vi "convertChannel.vi"(1 "Chn in":string) -> (0 "Chn out":string)   [LabVIEW 2023, in "ScopeNi.lvclass"]
uses:
  ScopeNi.lvclass
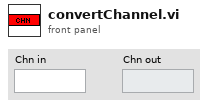
[diagram p1: front panel]
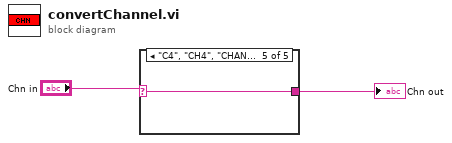
[diagram p0: block diagram]
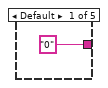
[diagram p2: hidden frame]
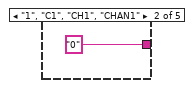
[diagram p3: hidden frame]
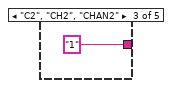
[diagram p4: hidden frame]
diagram:
  n1 = case shown="\"C4\", \"CH4\", \"CHAN4\"" "Chn in" {
    selector: "Chn in" -> [_ _ _ w6 w7]
    tunnel: ["0" "0" "1" w6 w7] -> w1
    frame Default {
    }
    frame "1", "C1", "CH1", "CHAN1" {
    }
    frame "C2", "CH2", "CHAN2" {
    }
    frame "C3", "CH3", "CHAN3" {
    }
    frame "C4", "CH4", "CHAN4" {
    }
  }
  "Chn out" <- w1
